vi "Triangle2Mesh.vi"(10 "Color":T1={"Alpha"=1.0, "Color"=0} {"Alpha" min=0.0 max=1.0 scale=0.0..1.0}, 11 "Triangles":T2[](array[typedef])) -> (3 "Refnum":refnum<vi>)   [LabVIEW 2014]
uses:
  TypeDefs/TriangleFace.ctl
  TypeDefs/Point3D.ctl
  TypeDefs/Color.ctl
  <vilib>/picture/3D Picture Control/NI_3D Picture Control.lvlib
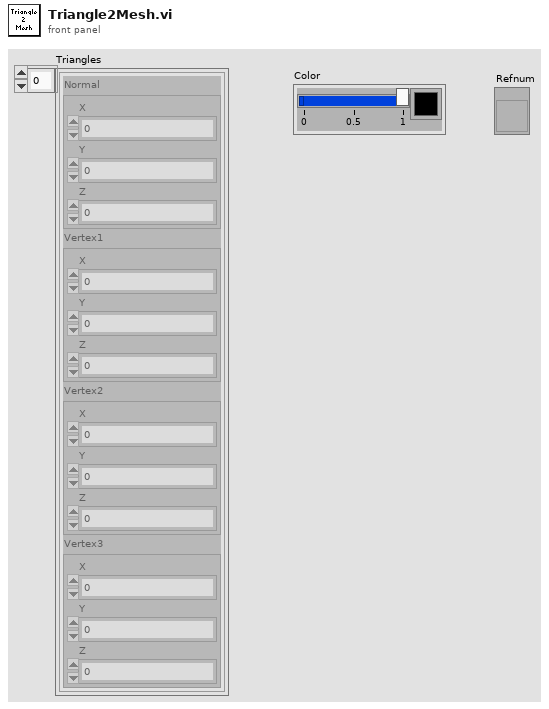
[diagram p1: front panel]
types:
  T1 = typedef "Color.ctl" = cluster{"Alpha":dbl, "Color":u32}
  T2 = typedef "TriangleFace.ctl" = cluster{"Normal":T3, "Vertex1":T3, "Vertex2":T3, "Vertex3":T3}
  T3 = typedef "Point3D.ctl" = cluster{"X":sgl, "Y":sgl, "Z":sgl}
  T4 = enum16{"Overall", "Per Primitive", "Per Vertex", "Binding Off"}
  T5 = enum16{"Points", "Lines", "Line Strip", "Line Loop", "Triangles", "Triangle Strip", "Triangle Fan", "Quads", "Quad Strip", "Polygon"}
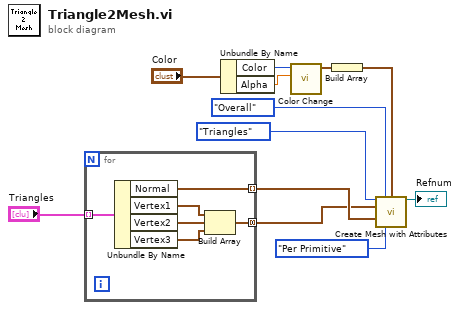
[diagram p0: block diagram]
diagram:
  n1 = for {
    tunnel: "Triangles" -> [w18] mode=indexing
    tunnel: [w14] -> w10 mode=concatenating
    tunnel: [w13] -> w11 mode=indexing
    n2 = Unbundle By Name(w18) -> ("Normal"=w13:T3, "Vertex1"=w17:T3, "Vertex2"=w16:T3, "Vertex3"=w15:T3)
    n3 = Build Array(w17, w16, w15) -> (w14:T3[])
  }
  n4 = Unbundle By Name("Color") -> ("Color"=w4:u32, "Alpha"=w3:dbl)
  n5 = call <vilib>:"Color Change.vi"("Alpha"=w3, "Color"=w4) -> ("RGBA"=w7:cluster{"R":sgl, "G":sgl, "B":sgl, "A":sgl})  [unwired: 9 in]
  n6 = Build Array(w7) -> (w6:cluster{"R":sgl, "G":sgl, "B":sgl, "A":sgl}[])
  n7 = call <vilib>:"Create Mesh with Attributes.vi"("Draw Mode"=T5."Triangles", "Color Binding Mode"=T4."Overall", "Color Array"=w6, "Vertex Array"=w10, "Normal Array"=w11, "Normal Binding Mode"=T4."Per Primitive") -> ("New Mesh Refnum"=→"Refnum":refnum<vi>)  [unwired: 8 in, 1 out]
